vi "GUI.vi"() -> ()   [LabVIEW 2023]
uses:
  <vilib>/userDefined/High Color/IMAQdx.ctl
  SM_GUI.ctl
  GV_obraz.vi
  GV_exit.vi
  Pulpit/GV_TakePhoto.vi
  GV_PickCam.vi
  GV_StartStop.vi
panel:
  in  "Select Camera:":T1
  out "Image":T2(plugin-control)
  in  "EXIT":bool
  in  "Enable TCP":bool
  in  "Take photo":bool
  in  "Stop":bool
  in  "Start":bool
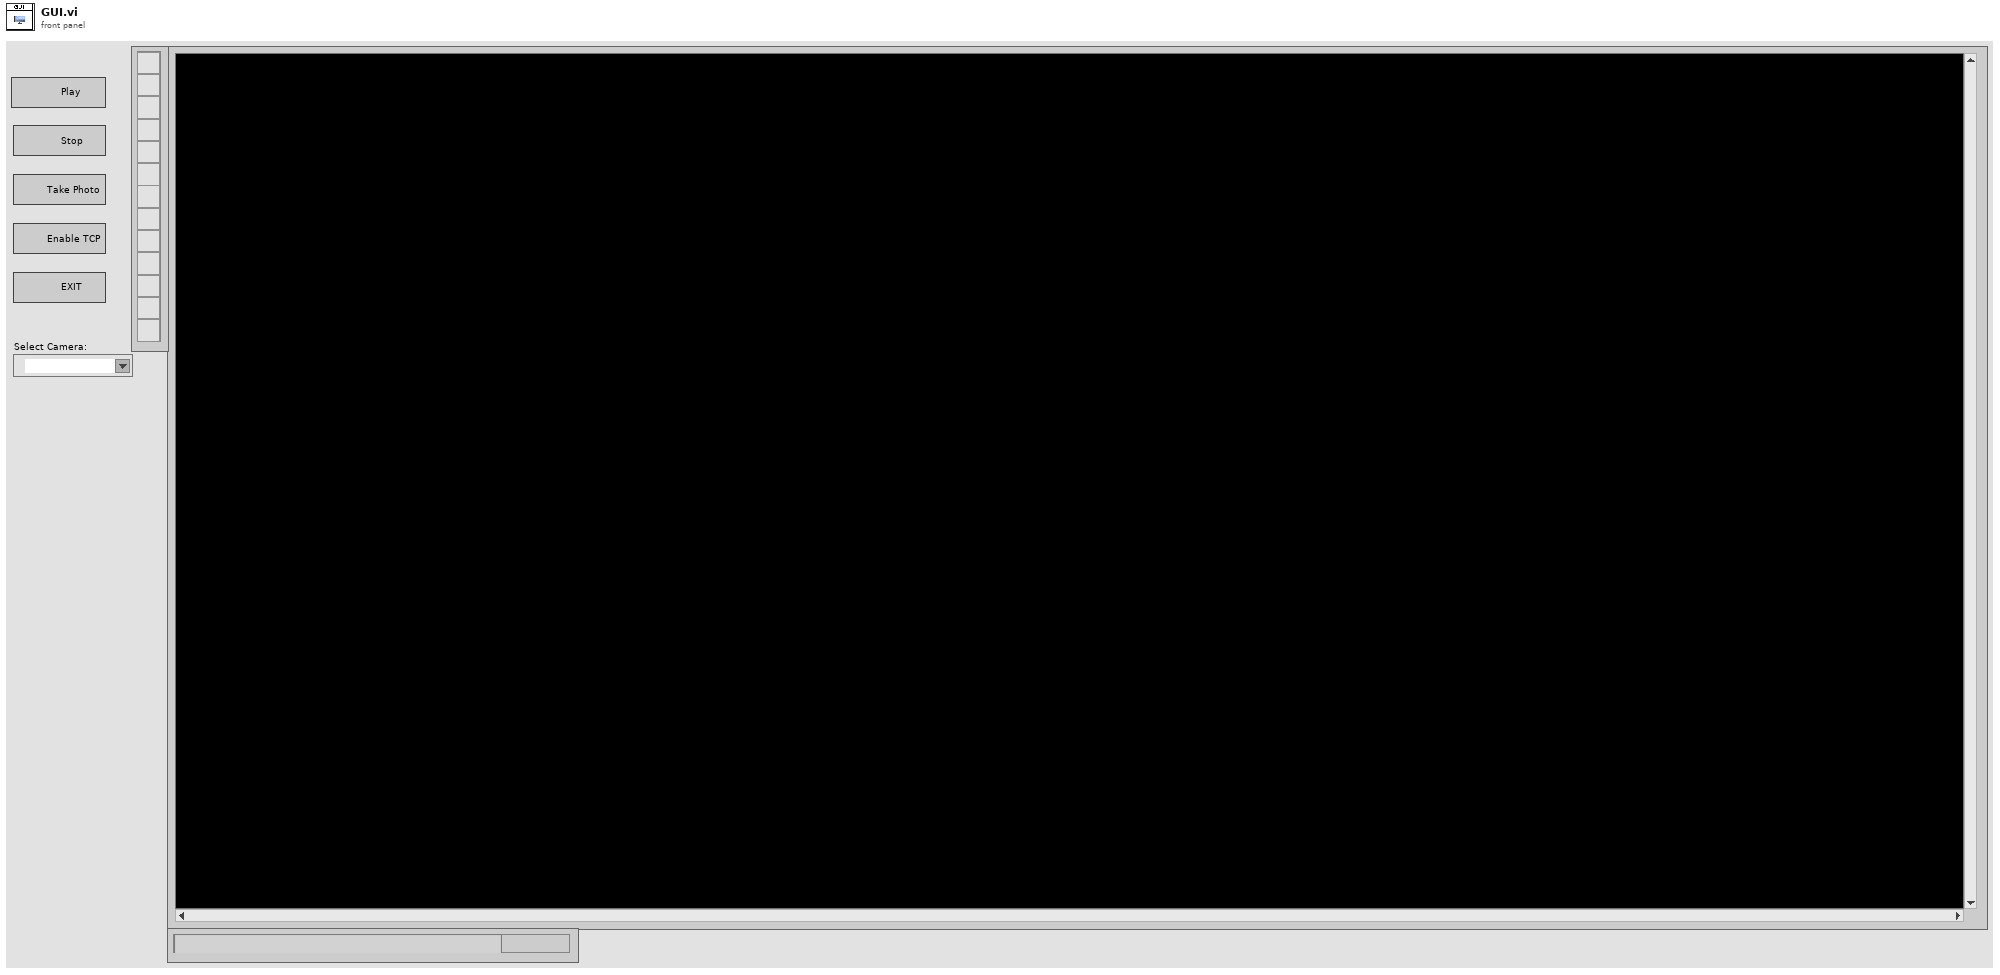
[diagram p1: front panel]
types:
  T1 = typedef "IMAQdx.ctl" = refnum<k21>
  T2 = typedef "IMAQ Image.ctl" = refnum<image>
  T3 = typedef "SM_GUI.ctl" = enum16{"Initialize", "Idle", "Start", "Stop", "Enable TCP", "Exit", ""}
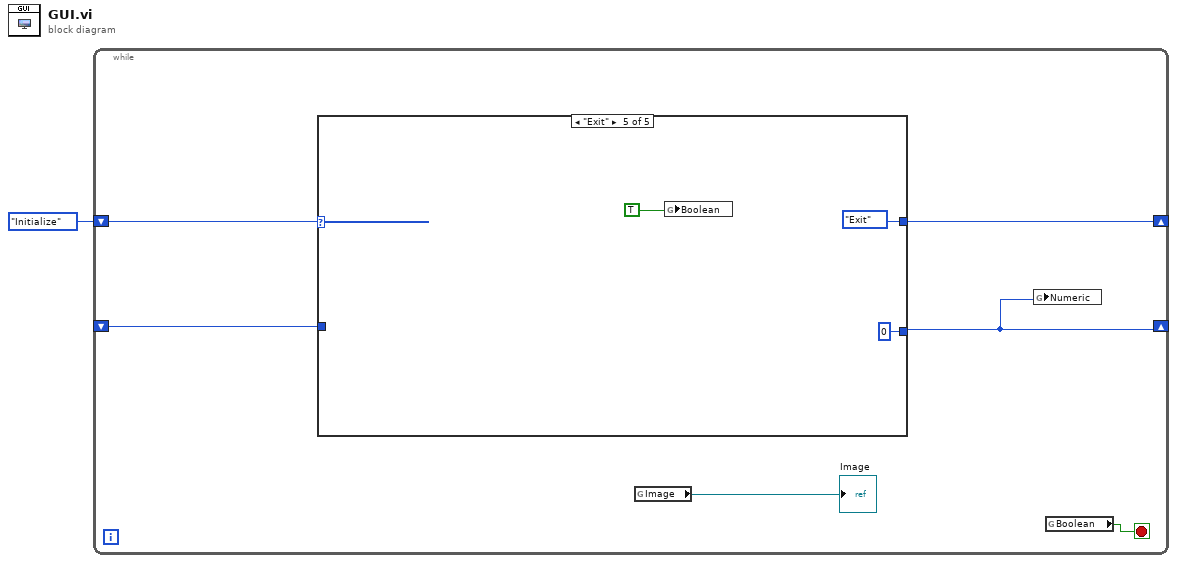
[diagram p0: block diagram]
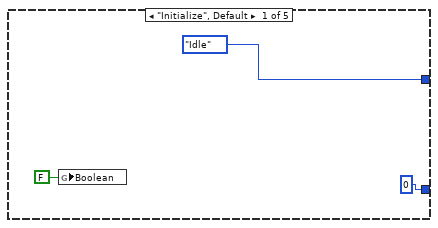
[diagram p2: hidden frame]
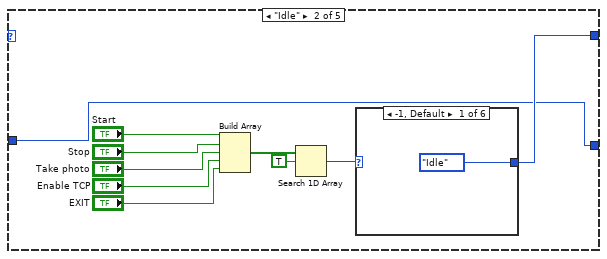
[diagram p3: hidden frame]
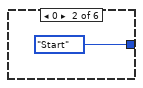
[diagram p4: hidden frame]
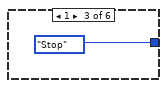
[diagram p5: hidden frame]
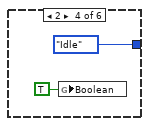
[diagram p6: hidden frame]
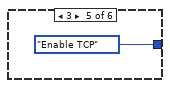
[diagram p7: hidden frame]
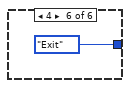
[diagram p8: hidden frame]
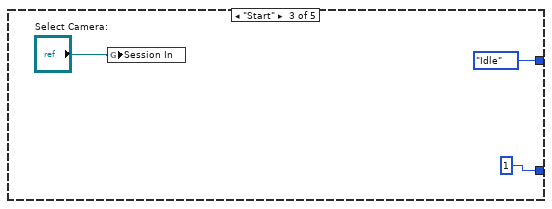
[diagram p9: hidden frame]
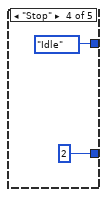
[diagram p10: hidden frame]
diagram:
  n1 = while {
    shift-right: [w5] -> _
    shift-left: SM_GUI."Initialize" ("SM_GUI_States") -> [w6]
    shift-right: [w3] -> _
    shift-left: _ -> [w4]
    stop <- w2 stop-if-true
    n2 = case shown="\"Exit\"" w6 {
      tunnel: [SM_GUI."Idle" ("SM_GUI_States") w13 SM_GUI."Idle" ("SM_GUI_States") SM_GUI."Idle" ("SM_GUI_States") SM_GUI."Exit" ("SM_GUI_States")] -> w5
      tunnel: w4 -> [_ w11 _ _ _]
      tunnel: [0 ("Numeric") w11 1 ("Numeric") 2 ("Numeric") 0 ("Numeric")] -> w3
      frame "Initialize", Default {
        n3 = global write "GV_exit.vi" "Boolean"(FALSE ("Boolean")) -> ()
      }
      frame "Idle" {
        n4 = Build Array("Start", "Stop", "Take photo", "Enable TCP", "EXIT") -> (w20:bool[])
        n5 = Search 1D Array(1D array=w20, element=TRUE) -> (index of element=w14:i32)  [unwired: 1 in]
        n6 = case shown="-1, Default" w14 {
          tunnel: [SM_GUI."Idle" ("SM_GUI_States") SM_GUI."Start" ("SM_GUI_States") SM_GUI."Stop" ("SM_GUI_States") SM_GUI."Idle" ("SM_GUI_States") SM_GUI."Enable TCP" ("SM_GUI_States") SM_GUI."Exit" ("SM_GUI_States")] -> w13
          frame -1, Default {
          }
          frame 0 {
          }
          frame 1 {
          }
          frame 2 {
            n7 = global write "GV_TakePhoto.vi" "Boolean"(TRUE ("Boolean")) -> ()
          }
          frame 3 {
          }
          frame 4 {
          }
        }
      }
      frame "Start" {
        n8 = global write "GV_PickCam.vi" "Session In"("Select Camera:") -> ()
      }
      frame "Stop" {
      }
      frame "Exit" {
        n9 = global write "GV_exit.vi" "Boolean"(TRUE ("Boolean")) -> ()
      }
    }
    n10 = global read "GV_obraz.vi" "Image"() -> (→"Image":T2)
    n11 = global write "GV_StartStop.vi" "Numeric"(w3) -> ()
    n12 = global read "GV_exit.vi" "Boolean"() -> (w2:bool)
  }
